vi "read_data.vi"(6 "Samples to Average":u32, 8 "error in (no error)":errorcluster, 9 "Read Period":dbl, 10 "Desired Data":string, 11 "VISA In":refnum<visa-resource-name>) -> (0 "error out":errorcluster, 1 "Series Cap Avg":dbl, 2 "Parallel Cap Avg":dbl, 3 "VISA Out":refnum<visa-resource-name>, 4 "Conductance Avg":dbl)   [LabVIEW 2011]
panel:
  out "Elapsed Time":dbl
  out "Conductance":dbl[](array[numeric])
  out "Serial Cap":dbl[](array[numeric])
  out "Parallel Cap":dbl[](array[numeric])
  out "Avg Count":u32
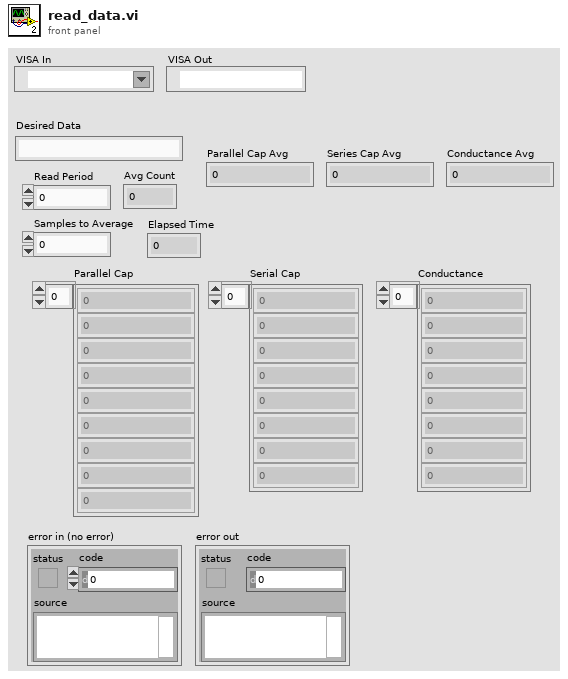
[diagram p1: front panel]
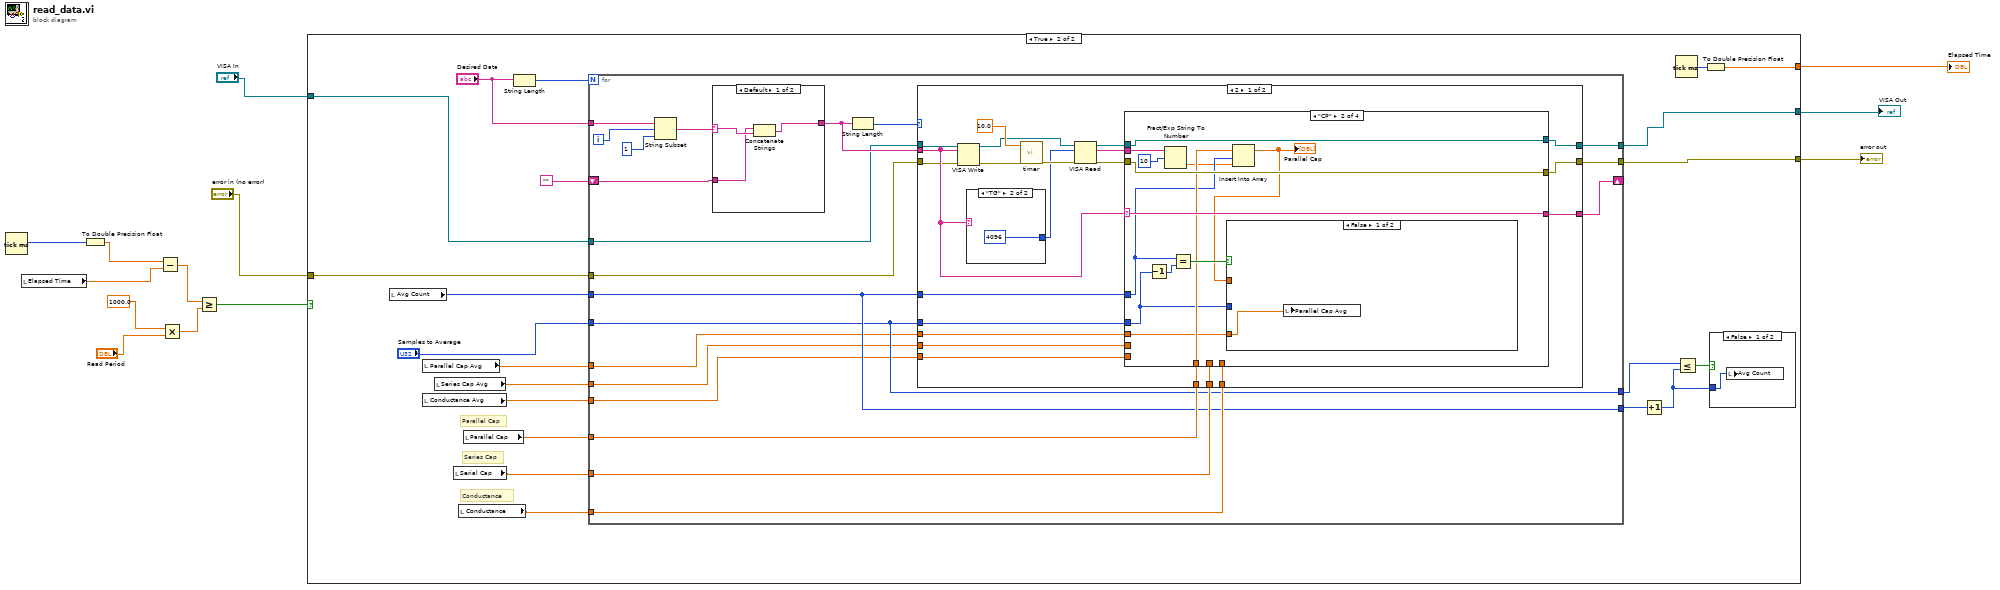
[diagram p0: block diagram]
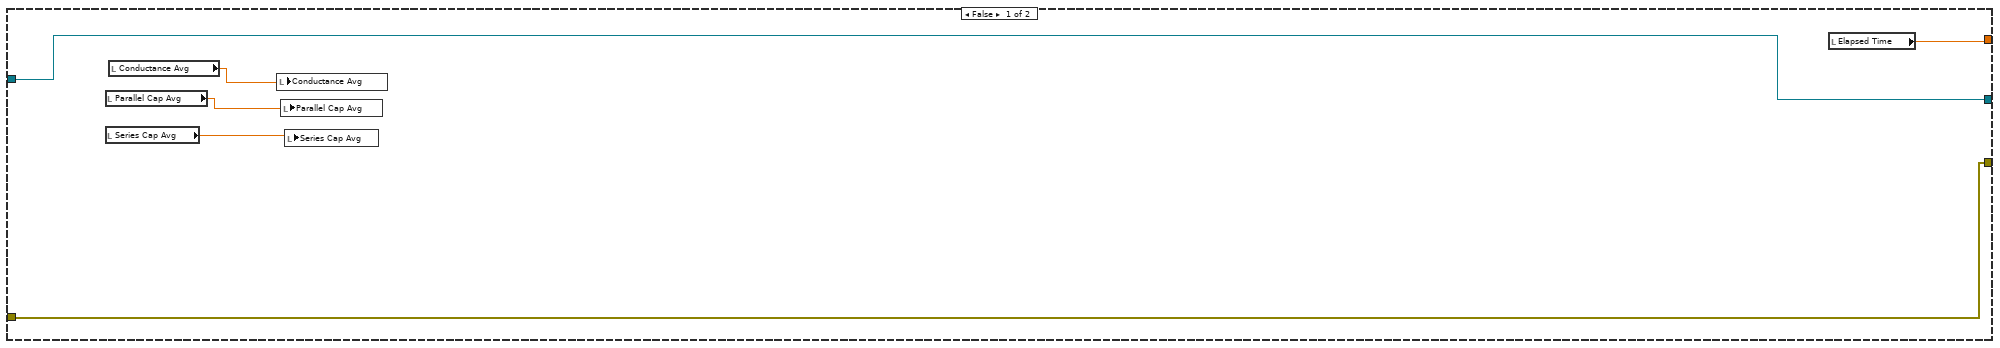
[diagram p2: hidden frame]
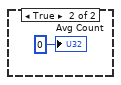
[diagram p3: hidden frame]
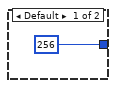
[diagram p4: hidden frame]
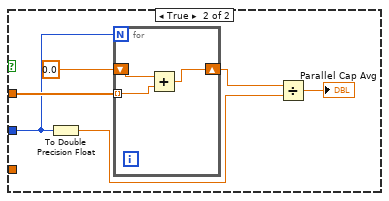
[diagram p6: hidden frame]
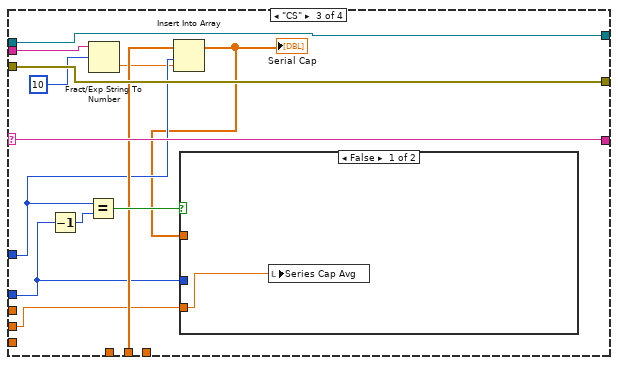
[diagram p7: hidden frame]
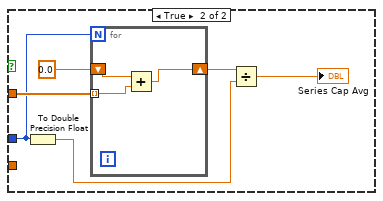
[diagram p8: hidden frame]
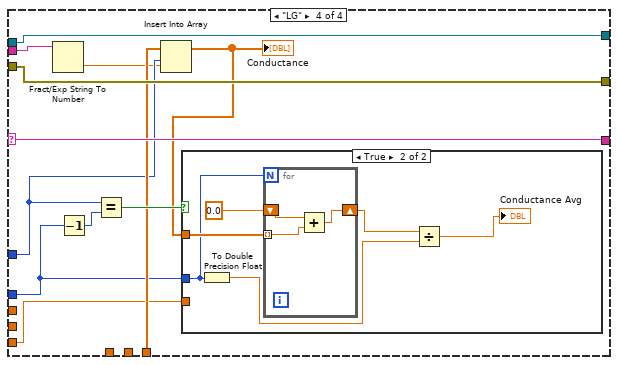
[diagram p9: hidden frame]
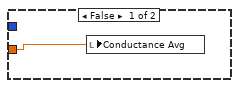
[diagram p10: hidden frame]
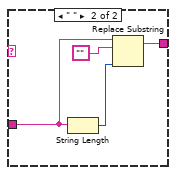
[diagram p12: hidden frame]
diagram:
  n1 = Tick Count (ms)() -> (millisecond timer value=w11:u32)
  n2 = local read "Elapsed Time"() -> (w10:dbl)
  n3 = To Double Precision Float(number=w11) -> (double precision float=w9:dbl)
  n4 = Subtract(x=w9, y=w10) -> (x-y=w6:dbl)
  n5 = Multiply(x=1000.0 ("y"), y="Read Period") -> (x*y=w5:dbl)
  n6 = Greater Or Equal?(x=w6, y=w5) -> (x >= y?=w7:bool)
  n7 = case shown="True" w7 {
    tunnel: [w19 w34] -> w8
    tunnel: [w14 w23] -> w4
    tunnel: [w15 w22] -> w3
    tunnel: "VISA In" -> [w15 w21]
    tunnel: "error in (no error)" -> [w14 w20]
    frame False {
      n8 = local read "Parallel Cap Avg"() -> (w17:dbl)
      n9 = local read "Series Cap Avg"() -> (w18:dbl)
      n10 = local read "Conductance Avg"() -> (w16:dbl)
      n11 = local write "Conductance Avg"(w16) -> ()
      n12 = local write "Parallel Cap Avg"(w17) -> ()
      n13 = local write "Series Cap Avg"(w18) -> ()
      n14 = local read "Elapsed Time"() -> (w19:dbl)
    }
    frame True {
      # "Conductance"
      # "Series Cap"
      # "Parallel Cap"
      n15 = local read "Avg Count"() -> (w37:u32)
      n16 = local read "Parallel Cap Avg"() -> (w25:dbl)
      n17 = local read "Conductance Avg"() -> (w24:dbl)
      n18 = local read "Series Cap Avg"() -> (w26:dbl)
      n19 = local read "Serial Cap"() -> (w31:dbl[])
      n20 = local read "Conductance"() -> (w30:dbl[])
      n21 = local read "Parallel Cap"() -> (w32:dbl[])
      n22 = String Length(string="Desired Data") -> (length=w33:i32)
      n23 = for {
        N: w33 -> [_]
        tunnel: "Desired Data" -> [w60]
        shift-right: [w50] -> _
        shift-left: "" -> [w59]
        tunnel: w21 -> [w55]
        tunnel: w20 -> [w54]
        tunnel: w32 -> [w51]
        tunnel: w31 -> [w52]
        tunnel: w30 -> [w53]
        tunnel: [w49] -> w22
        tunnel: [w48] -> w23
        tunnel: "Samples to Average" -> [w46]
        tunnel: w37 -> [w47]
        tunnel: [w47] -> w36
        tunnel: [w46] -> w28
        tunnel: w26 -> [w45]
        tunnel: w25 -> [w44]
        tunnel: w24 -> [w43]
        i -> [w62]
        n24 = String Subset(string=w60, offset (0)=w62, length (rest)=1 ("length (rest)")) -> (substring=w58:string)
        n25 = case shown="Default" w58 {
          selector: w58 -> [w162 _]
          tunnel: w59 -> [w161 w165]
          tunnel: [w163 w166] -> w56
          frame Default {
            n26 = Concatenate Strings(w161, w162) -> (w163:string)
          }
          frame " " {
            n27 = String Length(string=w165) -> (length=w164:i32)
            n28 = Replace Substring(2:w164, 4:"", 5:w165) -> (1:w166:string)  [unwired: 1 in, 1 out]
          }
        }
        n29 = String Length(string=w56) -> (length=w57:i32)
        n30 = case shown="2" w57 {
          tunnel: w56 -> [w75 w160]
          tunnel: w55 -> [w74 w158]
          tunnel: w54 -> [w73 w159]
          tunnel: w53 -> [w83 _]
          tunnel: w52 -> [w82 _]
          tunnel: w51 -> [w81 _]
          tunnel: [w80 w160] -> w50
          tunnel: [w78 w159] -> w48
          tunnel: [w79 w158] -> w49
          tunnel: w46 -> [w77 _]
          tunnel: w47 -> [w76 _]
          tunnel: w45 -> [w65 _]
          tunnel: w44 -> [w64 _]
          tunnel: w43 -> [w63 _]
          frame 2 {
            n31 = VISA Write(VISA resource name=w74, write buffer=w75, error in (no error)=w73) -> (VISA resource name out=w68:refnum<visa-resource-name>, error out=w72:errorcluster)  [unwired: 1 out]
            n32 = case shown="\"TG\"" w75 {
              tunnel: [256 u32 4096] -> w67
              frame Default {
              }
              frame "TG" {
              }
            }
            n33 = call "timer.vi"("error in (no error)"=w72, "Delay Time"=10.0) -> ("error out"=w69:errorcluster)  [unwired: 9 in]
            n34 = VISA Read(VISA resource name=w68, byte count=w67, error in (no error)=w69) -> (VISA resource name out=w71:refnum<visa-resource-name>, read buffer=w66:string, error out=w70:errorcluster)  [unwired: 1 out]
            n35 = case shown="\"CP\"" w75 {
              selector: w75 -> [w89 w100 w123 w145]
              tunnel: w71 -> [w88 w102 w125 w147]
              tunnel: w70 -> [w87 w101 w124 w146]
              tunnel: w83 -> [_ _ _ w143]
              tunnel: w82 -> [_ _ w121 _]
              tunnel: w81 -> [_ w98 _ _]
              tunnel: [w89 w100 w123 w145] -> w80
              tunnel: [w88 w102 w125 w147] -> w79
              tunnel: [w87 w101 w124 w146] -> w78
              tunnel: w77 -> [_ w94 w117 w140]
              tunnel: w76 -> [_ w97 w120 w142]
              tunnel: w66 -> [_ w93 w116 w138]
              tunnel: w65 -> [_ _ w114 _]
              tunnel: w64 -> [_ w91 _ _]
              tunnel: w63 -> [_ _ _ w136]
              frame Default {
              }
              frame "CP" {
                n36 = Decrement(x=w94) -> (x-1=w95:u32)
                n37 = Fract/Exp String To Number(string=w93, offset=10) -> (number=w92:dbl)  [unwired: 2 in, 1 out]
                n38 = Equal?(x=w97, y=w95) -> (x = y?=w99:bool)
                n39 = Insert Into Array(array=w98, index=w97, new element=w92) -> (w96:dbl[])
                "Parallel Cap" <- w96
                n40 = case shown="False" w99 {
                  tunnel: w96 -> [_ w105]
                  tunnel: w94 -> [_ w104]
                  tunnel: w91 -> [w103 _]
                  frame False {
                    n41 = local write "Parallel Cap Avg"(w103) -> ()
                  }
                  frame True {
                    n42 = To Double Precision Float(number=w104) -> (double precision float=w106:dbl)
                    n43 = for {
                      N: w104 -> [_]
                      tunnel: w105 -> [w111] mode=indexing
                      shift-right: [w110] -> w107
                      shift-left: 0.0 -> [w112]
                      n44 = Add(x=w112, y=w111) -> (x+y=w110:dbl)
                    }
                    n45 = Divide(x=w107, y=w106) -> (x/y=→"Parallel Cap Avg":dbl)
                  }
                }
              }
              frame "CS" {
                n46 = Decrement(x=w117) -> (x-1=w118:u32)
                n47 = Equal?(x=w120, y=w118) -> (x = y?=w122:bool)
                n48 = Fract/Exp String To Number(string=w116, offset=10) -> (number=w115:dbl)  [unwired: 2 in, 1 out]
                n49 = Insert Into Array(array=w121, index=w120, new element=w115) -> (w119:dbl[])
                "Serial Cap" <- w119
                n50 = case shown="False" w122 {
                  tunnel: w119 -> [_ w132]
                  tunnel: w117 -> [_ w127]
                  tunnel: w114 -> [w126 _]
                  frame False {
                    n51 = local write "Series Cap Avg"(w126) -> ()
                  }
                  frame True {
                    n52 = To Double Precision Float(number=w127) -> (double precision float=w129:dbl)
                    n53 = for {
                      N: w127 -> [_]
                      tunnel: w132 -> [w134] mode=indexing
                      shift-right: [w133] -> w130
                      shift-left: 0.0 -> [w135]
                      n54 = Add(x=w135, y=w134) -> (x+y=w133:dbl)
                    }
                    n55 = Divide(x=w130, y=w129) -> (x/y=→"Series Cap Avg":dbl)
                  }
                }
              }
              frame "LG" {
                n56 = Fract/Exp String To Number(string=w138) -> (number=w137:dbl)  [unwired: 3 in, 1 out]
                n57 = Decrement(x=w140) -> (x-1=w141:u32)
                n58 = Equal?(x=w142, y=w141) -> (x = y?=w144:bool)
                n59 = Insert Into Array(array=w143, index=w142, new element=w137) -> (w139:dbl[])
                "Conductance" <- w139
                n60 = case shown="True" w144 {
                  tunnel: w139 -> [_ w154]
                  tunnel: w140 -> [_ w149]
                  tunnel: w136 -> [w148 _]
                  frame False {
                    n61 = local write "Conductance Avg"(w148) -> ()
                  }
                  frame True {
                    n62 = To Double Precision Float(number=w149) -> (double precision float=w151:dbl)
                    n63 = for {
                      N: w149 -> [_]
                      tunnel: w154 -> [w156] mode=indexing
                      shift-right: [w155] -> w152
                      shift-left: 0.0 -> [w157]
                      n64 = Add(x=w157, y=w156) -> (x+y=w155:dbl)
                    }
                    n65 = Divide(x=w152, y=w151) -> (x/y=→"Conductance Avg":dbl)
                  }
                }
              }
            }
          }
          frame Default {
          }
        }
      }
      n66 = Increment(x=w36) -> (x+1=w27:u32)
      n67 = Tick Count (ms)() -> (millisecond timer value=w35:u32)
      n68 = Less Or Equal?(x=w28, y=w27) -> (x <= y?=w29:bool)
      n69 = To Double Precision Float(number=w35) -> (double precision float=w34:dbl)
      n70 = case shown="False" w29 {
        tunnel: w27 -> [w41 _]
        frame False {
          n71 = local write "Avg Count"(w41) -> ()
        }
        frame True {
          "Avg Count" <- u32 0 ("Avg Count")
        }
      }
    }
  }
  "Elapsed Time" <- w8
  "error out" <- w4
  "VISA Out" <- w3
